vi "CalculateMcsaHighRateFeatures.vi"(7 "motor informaiton":T1, 8 "error in (no error)":errorcluster, 9 "Map":T2, 10 "waveforms":waveform(sgl)[](array[waveform]), 11 "channels":T3[](array[typedef])) -> (0 "error out":errorcluster, 3 "channels out":T3[](array[typedef]))   [LabVIEW 2017, in "McsaAnalysisFunctions.lvlib"]
uses:
  <vilib>/addons/InsightCM/Utilities/Analysis/MCSA/McsaAnalysisFunctions.lvlib
  <vilib>/addons/InsightCM/Utilities/Analysis/MCSA/controls/McsaChannel.ctl
  <vilib>/addons/InsightCM/Utilities/Analysis/Shared/controls/Feature.ctl
  <vilib>/addons/InsightCM/Utilities/Analysis/Shared/controls/AmplitudeScale.ctl
  <vilib>/addons/InsightCM/MessageBus/Base/controls/KeyValuePair.ctl
  <vilib>/addons/PointValueMap/controls/PointMap.ctl
  <vilib>/addons/InsightCM/Utilities/Analysis/MCSA/controls/McsaMotor.ctl
  <vilib>/Analysis/5stat.llb/RMS (DBL).vi
  <vilib>/addons/PointValueMap/subVIs/Point_Write_double.vi
  <vilib>/addons/InsightCM/Utilities/MCSA/McsaUtilities.lvlib
  <vilib>/Analysis/NI_AALPro.lvlib
  <vilib>/addons/PointValueMap/PointValueMap.lvlib
  <vilib>/addons/InsightCM/Utilities/Analysis/Shared/AnalysisHelper.lvlib
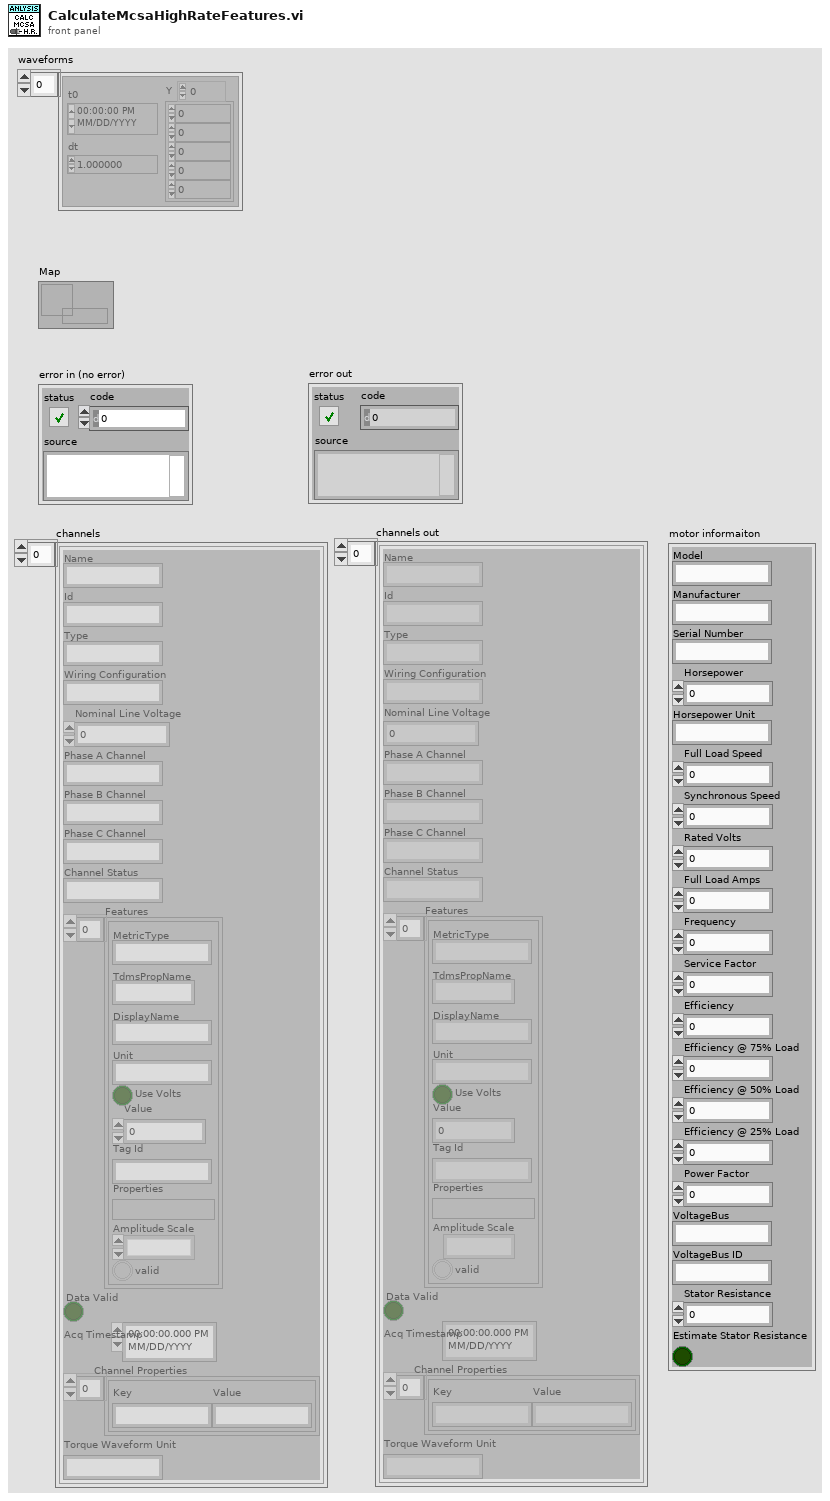
[diagram p1: front panel]
types:
  T1 = typedef "McsaAnalysisFunctions.lvlib/McsaMotor.ctl" = cluster{"Model":string, "Manufacturer":string, "Serial Number":string, "Horsepower":dbl, "Horsepower Unit":string, "Full Load Speed":dbl, "Synchronous Speed":dbl, "Rated Volts":dbl, "Full Load Amps":dbl, "Frequency":dbl, "Service Factor":dbl, "Efficiency":dbl, "Efficiency @ 75% Load":dbl, "Efficiency @ 50% Load":dbl, "Efficiency @ 25% Load":dbl, "Power Factor":dbl, "VoltageBus":string, "VoltageBus ID":string, "Stator Resistance":dbl, "Estimate Stator Resistance":bool}
  T2 = typedef "PointValueMap.lvlib/PointMap.ctl" = refnum<data-value>
  T3 = typedef "McsaAnalysisFunctions.lvlib/McsaChannel.ctl" = cluster{"Name":string, "Id":string, "Type":string, "Wiring Configuration":string, "Nominal Line Voltage":dbl, "Phase A Channel":string, "Phase B Channel":string, "Phase C Channel":string, "Channel Status":string, "Features":T4[], "Data Valid":bool, "Acq Timestamp":timestamp, "Channel Properties":T6[], "Torque Waveform Unit":string}
  T4 = typedef "AnalysisHelper.lvlib/Feature.ctl" = cluster{"MetricType":string, "TdmsPropName":string, "DisplayName":string, "Unit":string, "Use Volts":bool, "Value":dbl, "Tag Id":string, "Properties":variant, "Amplitude Scale":T5, "valid":bool}
  T5 = typedef "AnalysisHelper.lvlib/AmplitudeScale.ctl" = enum16{"rms", "peak", "pk-pk"}
  T6 = typedef "KeyValuePair.ctl" = cluster{"Key":string, "Value":string}
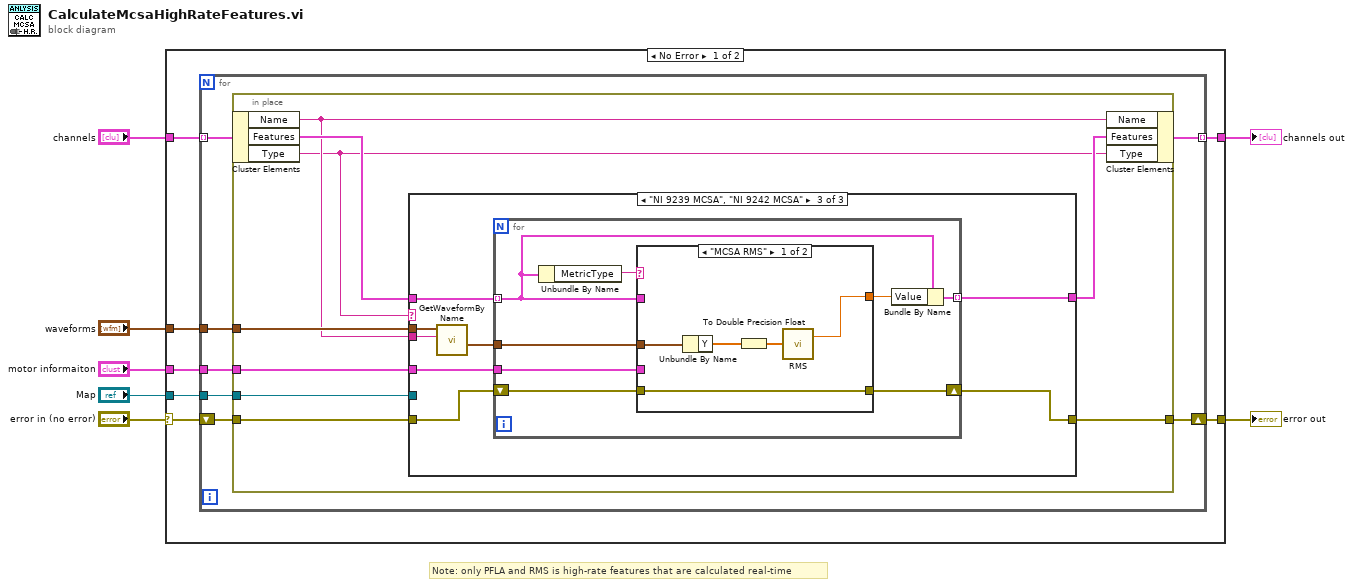
[diagram p0: block diagram]
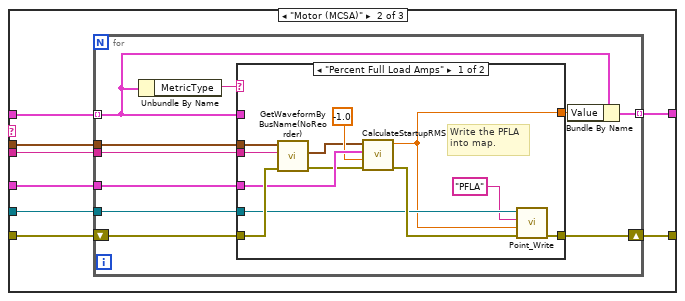
[diagram p3: hidden frame]
diagram:
  # "Note: only PFLA and RMS is high-rate features that are calculated real-time"
  n1 = case shown="No Error" "error in (no error)" {
    selector: "error in (no error)" -> [w14 w86]
    tunnel: [w10 w86] -> w7
    tunnel: "channels" -> [w11 w87]
    tunnel: [w12 w87] -> w5
    tunnel: "waveforms" -> [w13 _]
    tunnel: "Map" -> [w9 _]
    tunnel: "motor informaiton" -> [w8 _]
    frame No Error {
      n2 = for {
        tunnel: w11 -> [w17] mode=indexing
        tunnel: [w21] -> w12 mode=indexing
        tunnel: w13 -> [w18]
        shift-right: [w19] -> w10
        shift-left: w14 -> [w20]
        tunnel: w9 -> [w16]
        tunnel: w8 -> [w15]
        n3 = in-place {
          in-place-border: w20 -> [w26]
          in-place-border: [w30] -> w19
          in-place-border: w18 -> [w25]
          in-place-border: w15 -> [w29]
          in-place-border: w16 -> [w22]
          n4 = in-place-cluster #1(w17) -> ("Name"=w24:string, "Features"=w28:T4[], "Type"=w23:string)
          n5 = case shown="\"NI 9239 MCSA\", \"NI 9242 MCSA\"" w23 {
            tunnel: [w31 w40 w71] -> w27
            tunnel: w26 -> [w32 w39 w70]
            tunnel: w28 -> [w31 w38 w69]
            tunnel: w25 -> [_ w37 w66]
            tunnel: [w32 w36 w68] -> w30
            tunnel: w29 -> [_ w35 w67]
            tunnel: w24 -> [_ w34 w65]
            tunnel: w22 -> [_ w33 _]
            frame Default {
            }
            frame "Motor (MCSA)" {
              n6 = for {
                tunnel: w38 -> [w44] mode=indexing
                tunnel: [w50] -> w40 mode=indexing
                tunnel: w37 -> [w46]
                tunnel: w35 -> [w45]
                shift-right: [w48] -> w36
                shift-left: w39 -> [w49]
                tunnel: w34 -> [w42]
                tunnel: w33 -> [w41]
                n7 = Unbundle By Name(w44) -> ("MetricType"=w43:string)
                n8 = case shown="\"Percent Full Load Amps\"" w43 {
                  tunnel: [w53 _] -> w47
                  tunnel: w49 -> [w61 w63]
                  tunnel: [w56 w63] -> w48
                  tunnel: w46 -> [w62 _]
                  tunnel: w45 -> [w60 _]
                  tunnel: w44 -> [_ _]
                  tunnel: w42 -> [w52 _]
                  tunnel: w41 -> [w54 _]
                  frame "Percent Full Load Amps" {
                    # "Write the PFLA\ninto map."
                    n9 = call <vilib>:"GetWaveformByBusName(NoReorder).vi"("error in (no error)"=w61, "Bus Name"=w52, "Acq Waveforms"=w62) -> ("error out"=w58:errorcluster, "Waveform of Bus"=w57:waveform(dbl)[])  [unwired: 6 in, 1 out]
                    n10 = call <vilib>:"CalculateStartupRMS.vi"("error in (no error)"=w58, "frequency"=-1.0, "Motor"=w60, "current waveforms"=w57) -> ("error out"=w55:errorcluster, "Percent Full Load Amps [%FLA]"=w53:dbl)  [unwired: 6 in]
                    n11 = call-poly <vilib>:"Point_Write.vi"("Error In"=w55, "Value"=w53, "Tag"="PFLA", "Map"=w54) -> ("Error Out"=w56:errorcluster)  [unwired: 6 in, 1 out]
                  }
                  frame Default {
                  }
                }
                n12 = Bundle By Name(cluster=w44, "Value"=w47) -> (w50:T4)
              }
            }
            frame "NI 9239 MCSA", "NI 9242 MCSA" {
              n13 = call <vilib>:"GetWaveformByName.vi"("Channel Name"=w65, "Acq Waveforms"=w66) -> ("Waveform"=w64:waveform(sgl))  [unwired: 6 in, 3 out]
              n14 = for {
                tunnel: w69 -> [w74] mode=indexing
                tunnel: [w79] -> w71 mode=indexing
                tunnel: w67 -> [w75]
                shift-right: [w77] -> w68
                shift-left: w70 -> [w78]
                tunnel: w64 -> [w72]
                n15 = Unbundle By Name(w74) -> ("MetricType"=w73:string)
                n16 = case shown="\"MCSA RMS\"" w73 {
                  tunnel: [w81 _] -> w76
                  tunnel: w78 -> [w80 w85]
                  tunnel: [w80 w85] -> w77
                  tunnel: w75 -> [_ _]
                  tunnel: w74 -> [_ _]
                  tunnel: w72 -> [w82 _]
                  frame "MCSA RMS" {
                    n17 = Unbundle By Name(w82) -> ("Y"=w83:sgl[])
                    n18 = To Double Precision Float(number=w83) -> (double precision float=w84:dbl[])
                    n19 = call-poly <vilib>:"RMS.vi"("X"=w84) -> ("rms value"=w81:dbl)  [unwired: 1 out]
                  }
                  frame Default {
                  }
                }
                n20 = Bundle By Name(cluster=w74, "Value"=w76) -> (w79:T4)
              }
            }
          }
          n21 = in-place-cluster #1("Name"=w24, "Features"=w27, "Type"=w23) -> (w21:T3)
        }
      }
    }
    frame Error {
    }
  }
  "error out" <- w7
  "channels out" <- w5
